vi "niUSRP Tx Continuous Lab copy2.vi"() -> ()   [LabVIEW 2014]
uses:
  <vilib>/measure/maspectr.llb/FFT Power Spectrum and PSD for 1 Chan (CDB).vi
  <instrlib>/niUSRP/niUSRP Write Tx Data (CDB).vi
  <vilib>/measure/NI_MAPro.lvlib
  <vilib>/measure/NI_MABase.lvlib
panel:
  out "Waveform Graph":waveform(dbl)[](graph)
  in  "Stop Button":bool
  out "Frequency Plot":cluster{"f0":dbl, "df":dbl, "magnitude":dbl[]}(graph)
  out "IQ Plot":waveform(dbl)[](graph)
  in  "device name":refnum<k15>="192.168.10.2"
  out "Error Out":errorcluster
  in  "active antenna":string="TX/RX"
  in  "tone frequency":dbl=10000.0 format="%#_6p"
  in  "waveform size":dbl=10000.0
  out "Gain [dB] (actual)":dbl format="%#.6p"
  out "Carrier Frequency \n[Hz] (actual)":dbl=2450000000.0 format="%#.6p"
  out "IQ Sampling\nRate [s/sec] (actual)":dbl=10000000.0 format="%#.6p"
  in  "Gain [dB]":dbl format="%#.6p"
  in  "Carrier\nFrequency [Hz]":dbl=915000000.0 format="%#.6p"
  in  "IQ Sampling\nRate [s/sec]":dbl=10000000.0 format="%#.6p"
  # "IQ Transmitter"
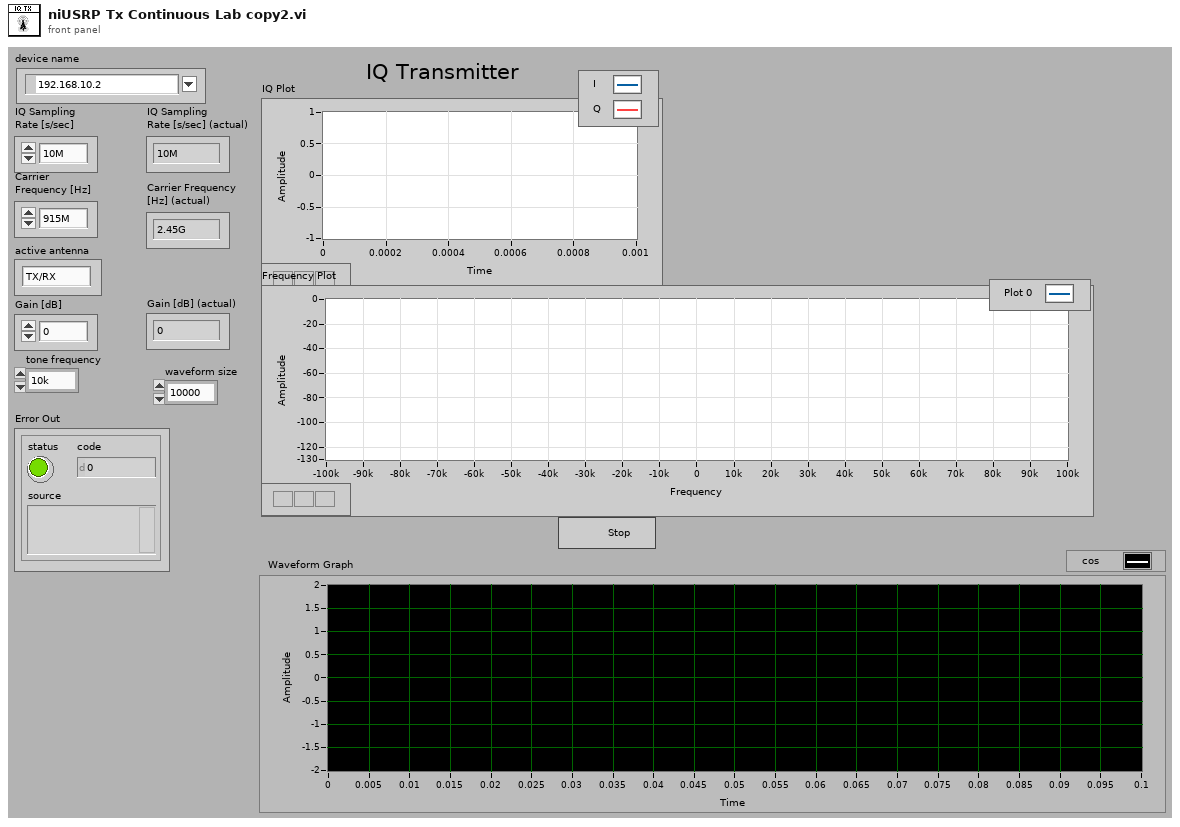
[diagram p1: front panel]
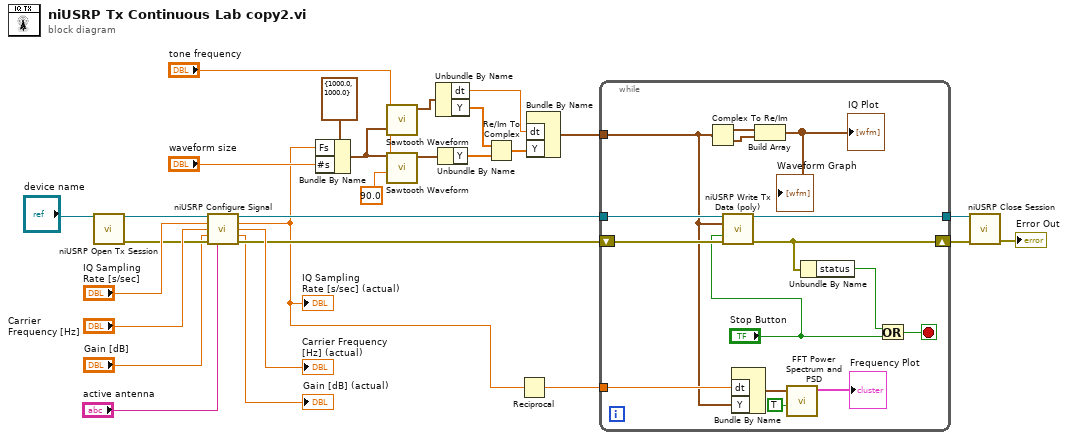
[diagram p0: block diagram]
diagram:
  n1 = call <instrlib>:"niUSRP Open Tx Session.vi"("device names"="device name") -> ("session handle out"=w28:refnum<k15>, "error out"=w25:errorcluster)  [unwired: 13 in]
  n2 = call <instrlib>:"niUSRP Configure Signal.vi"("session handle"=w28, "IQ rate"="IQ Sampling\nRate [s/sec]", "carrier frequency"="Carrier\nFrequency [Hz]", "gain"="Gain [dB]", "error in (no error)"=w25, "active antenna"="active antenna") -> ("session handle out"=w23:refnum<k15>, "coerced IQ rate"=w5:dbl, "coerced carrier frequency"=→"Carrier Frequency \n[Hz] (actual)":dbl, "coerced gain"=→"Gain [dB] (actual)":dbl, "error out"=w22:errorcluster)  [unwired: 5 in]
  "IQ Sampling\nRate [s/sec] (actual)" <- w5
  n3 = Bundle By Name(cluster=cluster{"Fs":dbl, "#s":dbl} {"Fs"=1000.0, "#s"=1000.0} ("sampling info"), "Fs"=w5, "#s"="waveform size") -> (w17:cluster{"Fs":dbl, "#s":dbl})
  n4 = call <vilib>:"Sawtooth Waveform.vi"("sampling info"=w17, "frequency"="tone frequency") -> ("signal out"=w13:waveform(dbl))  [unwired: 8 in, 1 out]
  n5 = call <vilib>:"Sawtooth Waveform.vi"("sampling info"=w17, "phase"=90.0, "frequency"="tone frequency") -> ("signal out"=w14:waveform(dbl))  [unwired: 7 in, 1 out]
  n6 = Unbundle By Name(w13) -> ("dt"=w3:dbl, "Y"=w12:dbl[])
  n7 = Unbundle By Name(w14) -> ("Y"=w11:dbl[])
  n8 = Re/Im To Complex(1:w11, 2:w12) -> (0:w2:cdb[])
  n9 = Reciprocal(x=w5) -> (1/x=w6:dbl)
  n10 = Bundle By Name("dt"=w3, "Y"=w2) -> (w1:waveform(cdb))  [unwired: 1 in]
  n11 = while {
    tunnel: w23 -> [w41]
    tunnel: [w39] -> w21
    shift-right: [w38] -> w20
    shift-left: w22 -> [w40]
    tunnel: w1 -> [w30]
    tunnel: w6 -> [w34]
    stop <- w43 stop-if-true
    n12 = Complex To Re/Im(x + iy=w30) -> (x=w35:waveform(dbl), y=w36:waveform(dbl))
    n13 = call-poly <instrlib>:"niUSRP Write Tx Data (poly).vi"("session handle"=w41, "data"=w30, "end of data?"="Stop Button", "error in (no error)"=w40) -> ("session handle out"=w39:refnum<k15>, "error out"=w38:errorcluster)  [unwired: 10 in]
    n14 = Bundle By Name("dt"=w34, "Y"=w30) -> (w37:waveform(cdb))  [unwired: 1 in]
    n15 = Build Array(w35, w36) -> (→"IQ Plot" →"Waveform Graph":waveform(dbl)[])
    n16 = call-poly <vilib>:"FFT Power Spectrum and PSD.vi"("dB On (F)"=TRUE, "time signal"=w37) -> ("Power Spectrum / PSD"=→"Frequency Plot":cluster{"f0":dbl, "df":dbl, "magnitude":dbl[]})  [unwired: 6 in, 3 out]
    n17 = Unbundle By Name(w38) -> ("status"=w42:bool)
    n18 = Or(x=w42, y="Stop Button") -> (x .or. y?=w43:bool)
  }
  n19 = call <instrlib>:"niUSRP Close Session.vi"("session handle"=w21, "error in (no error)"=w20) -> ("error out"=→"Error Out":errorcluster)  [unwired: 13 in]
